vi "sig.handle_stop_lua.vi"(5 "LuaVIEW reference":T1) -> (15 "error out":errorcluster)   [LabVIEW 2012]
doc: "Handle the stop signal. When a task starts, the handling of the stop signal is delegated to a built-in mechanism that interrupts the task and runs any cleanup functions before terminating the virtual machine. This function disables built in handling and therefore obliges your script to perform custom handling of the stop signal. Custom handling is rarely useful. If your task manages resources that must be freed before the task is terminated, adding cleanup functions using \"lv.addcleanup()\" is more convenient and safer because cleanup functions are not skipped when an error occurs.\n\nThe only situation that custom stop handling can cover that cleanup functions cannot is when the task must verify whether stopping is allowed, and resume the script when it is not. When the condition that makes stopping impossible is a result of the script execution instead of some external asynchronous event, it is possible to use \"sig.disallow_stop()\" instead, which is neater since it can be placed close to the code that should not be interrupted and has as advantage that the task manager \"stop\" button is greyed to make explicit that the task is not in a stoppable condition.\nErrors:\nFunction must be called from a task context but was not."
uses:
  typedefs/t_LuaVIEW Reference.ctl
  typedefs/t_LuaVIEW Task Signals.ctl
  typedefs/t_LuaVIEW Task State Methods.ctl
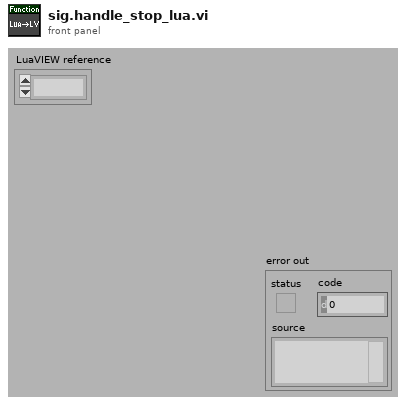
[diagram p1: front panel]
types:
  T1 = typedef "t_LuaVIEW Reference.ctl" = refnum<k1>
  T2 = typedef "t_LuaVIEW Task State Methods.ctl" = enum16{"cleanup", "set initial", "set mode", "set active mode", "set error", "get task info", "get script info", "set signal", "clear signal", "test handled", "test delegated", "test signal", "handle signal", "delegate signal", "allow signal", "disallow signal", "disallow all", "signals?", "delegated signals?", "protection++", "protection--", "protection=0", "message", "next message", "pop message", "message available?", "force stop", "set swap preps", "apply swap preps"}
  T3 = typedef "t_LuaVIEW Task Signals.ctl" = enum32{"resume", "pause", "swap", "stop", "confirm"}
  T4 = typedef "t_LuaVIEW Task State Pane.ctl" = refnum<vi>
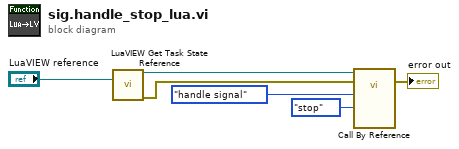
[diagram p0: block diagram]
diagram:
  n1 = call "LuaVIEW Get Task State Reference.vi"("LuaVIEW reference in"="LuaVIEW reference") -> ("task state reference"=w5:T4, "error out"=w1:errorcluster)  [unwired: 12 in, 1 out]
  n2 = call-by-ref "?"(reference=w5, error in=w1, "method"=t_LuaVIEW_Task_State_Methods."handle signal", "signal"=t_LuaVIEW_Task_Signals."stop") -> (error out=→"error out":errorcluster)  [unwired: 9 in, 6 out]
